vi "robot_const.vi"() -> ()   [LabVIEW 2014]
panel:
  in  "Tab Control":enum32{"Dimensions", "Misc."}(tab)
  in  "Height":dbl min=0.0 step=0.01
  in  "Length":dbl min=0.0 step=0.01
  in  "Width":dbl min=0.0 step=0.01
  # "Global Robot Constants"
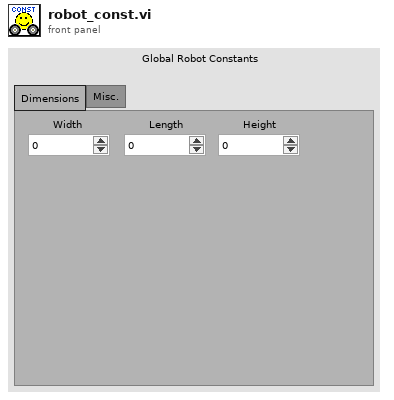
[diagram p1: front panel]
diagram:
